vi "Measure.vi"(8 "error in":errorcluster, 11 "4081 in":refnum<class "4081.lvclass">) -> (0 "error out":errorcluster, 3 "4081 out":refnum<class "4081.lvclass">)   [LabVIEW 2019, in "4081.lvlib" / "4081.lvclass"]
uses:
  Library/4081.lvclass
  C:/Users/Public/Documents/Development/builds/Instruments/Instruments.lvlibp/Library/Instruments.lvclass
  builds/Instruments/Instruments.lvlibp/Accessors/Write Measured.vi
  builds/Instruments/Multimeter.lvlibp/Library/Multimeter.lvclass
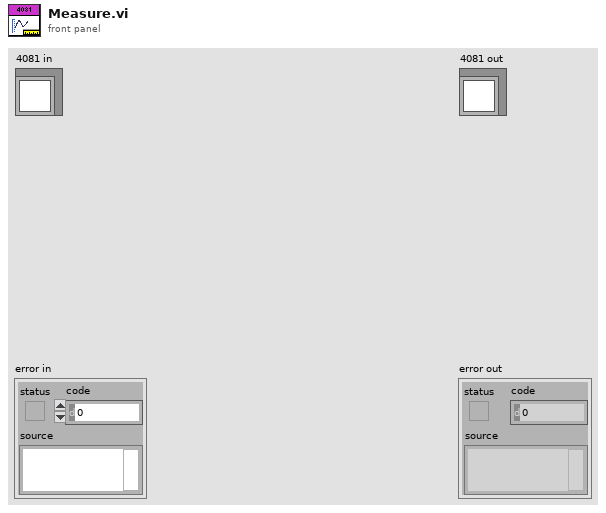
[diagram p1: front panel]
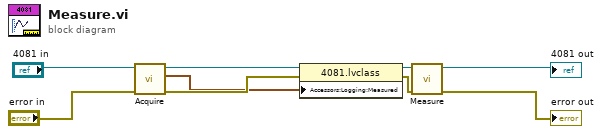
[diagram p0: block diagram]
diagram:
  n1 = call "Acquire.vi"("error in"="error in", "4081 in"="4081 in") -> ("error out"=w2:errorcluster, "Acquired"=w1:waveform(dbl)[], "4081 out"=w3:refnum<class "4081.lvclass">)  [unwired: 7 in]
  n2 = property class="4081.lvclass"(reference=w3, error in=w2, "Accessors:Logging:Measured"=w1) -> (reference out=w7:refnum<class "4081.lvclass">, error out=w6:errorcluster)
  n3 = call-parent "Measure.vi"("error in"=w6, "Multimeter in"=w7) -> ("error out"=→"error out":errorcluster, "Multimeter out"=→"4081 out":refnum<class "4081.lvclass">)  [unwired: 8 in]
